vi "cvt tag to tag bus tag.vi"(11 "CVT Tags":T1[](array[typedef])) -> (3 "TB Tags":refnum<class "tag descriptor.lvclass">[](array[class]))   [LabVIEW 2018, in "CVT configuration.lvclass"]
uses:
  CVT configuration.lvclass
  <vilib>/NI/Current Value Table/Type Defs/Data Types.ctl
  <vilib>/NI/Current Value Table/Current Value Table.lvlib
  <vilib>/NI/Current Value Table/Type Defs/Single Tag.ctl
  <vilib>/NI/Tag Bus/tag/tag descriptor.lvclass
panel:
  # "ADSFASDFASDFASDFASDFASD"
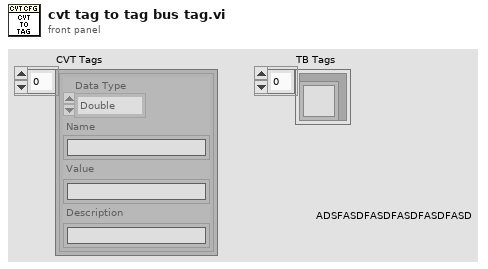
[diagram p1: front panel]
types:
  T1 = typedef "Current Value Table.lvlib/Single Tag.ctl" = cluster{"Data Type":T2, "Name":string, "Value":string, "Description":string}
  T2 = typedef "Current Value Table.lvlib/Data Types.ctl" = enum16{"Double", "Single", "I64", "I32", "I16", "I8", "U64", "U32", "U16", "U8", "String", "Boolean", "Array of U8", "Array of U16", "Array of U32", "Array of U64", "Array of I64", "Array of I32", "Array of I16", "Array of I8", "Array of Double", "Array of Single", "Array of Boolean", "Array of String"}
  T3 = typedef "tag bus.lvlib/tag descriptor.lvclass/Data Type.ctl" = enum16{"Double", "Single", "I64", "I32", "I16", "I8", "U64", "U32", "U16", "U8", "Boolean", "String", "Array of Double", "Array of Single", "Array of I64", "Array of I32", "Array of I16", "Array of I8", "Array of U64", "Array of U32", "Array of U16", "Array of U8", "Array of Boolean", "Array of String"}
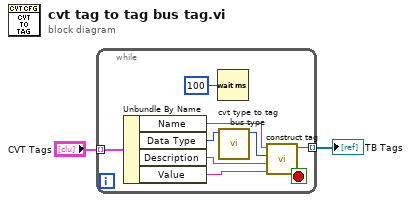
[diagram p0: block diagram]
diagram:
  n1 = while {
    tunnel: "CVT Tags" -> [w10] mode=indexing
    tunnel: [w8] -> w1 mode=indexing
    stop <- _ stop-if-true
    n2 = Unbundle By Name(w10) -> ("Name"=w7:string, "Data Type"=w9:T2, "Description"=w5:string, "Value"=w4:string)
    n3 = Wait (ms)(milliseconds to wait=u32 100) -> ()  [unwired: 1 out]
    n4 = call "cvt type to tag bus type.vi"("cvt type"=w9) -> ("Data Type"=w6:T3)  [unwired: 10 in]
    n5 = call <vilib>:"construct tag.vi"("raw default"=w4, "metadata"=w5, "data type"=w6, "name"=w7) -> ("system tag out"=w8:refnum<class "tag descriptor.lvclass">)  [unwired: 6 in, 1 out]
  }
  "TB Tags" <- w1
